vi "7HP_Process.vi"(0 "All samples in":sgl[][](array[numeric]), 1 "Serial number":u32, 2 "7HP Ch No":i16[](array[numeric]), 3 "Analysis info Index":i32[](array[numeric]), 4 "Probe Number":i32, 5 "Sampling Rate":dbl) -> ()   [LabVIEW 2021]
uses:
  <vilib>/Analysis/NI_AALBase.lvlib
  <vilib>/Analysis/baseanly.llb/Mean (DBL).vi
  Sub_vis/Upload Data.ctl
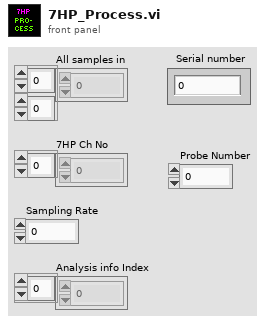
[diagram p1: front panel]
types:
  T1 = typedef "Upload Data.ctl" = enum16{"Voltage Array", "Time Trace Cluster"}
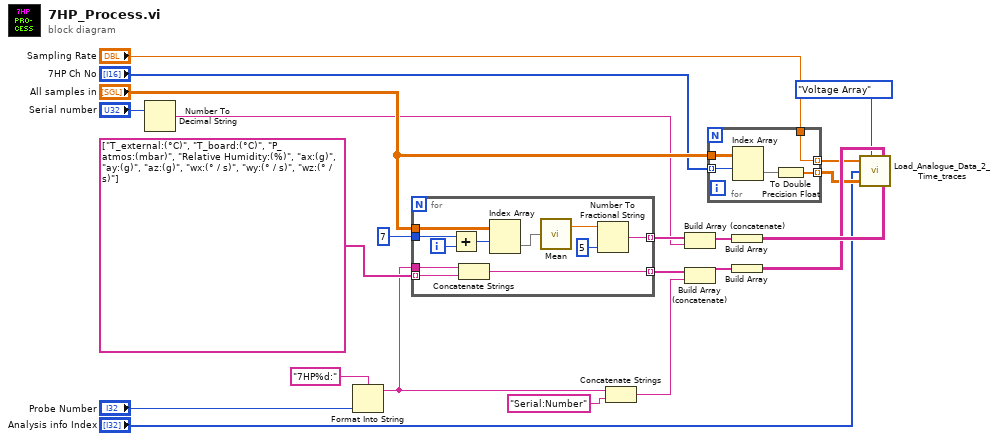
[diagram p0: block diagram]
diagram:
  n1 = Number To Decimal String(number="Serial number") -> (decimal integer string=w4:string)  [unwired: 1 in]
  n2 = Format Into String(format string="7HP%d:", "Probe Number") -> (resulting string=w9:string)  [unwired: 2 in, 1 out]
  n3 = for {
    tunnel: "All samples in" -> [w33]
    tunnel: 7 -> [w31]
    tunnel: w9 -> [w29]
    tunnel: string[] ["T_external:(°C)", "T_board:(°C)", "P_atmos:(mbar)", "Relative Humidity:(%)", "ax:(g)", "ay:(g)", "az:(g)", "wx:(° / s)", "wy:(° / s)", "wz:(° / s)"] -> [w28] mode=indexing
    tunnel: [w23] -> w10 mode=indexing
    tunnel: [w24] -> w7 mode=indexing
    i -> [w32]
    n4 = Add(x=w31, y=w32) -> (x+y=w30:i32)
    n5 = Concatenate Strings(w29, w28) -> (w24:string)
    n6 = Index Array(array=w33, index (row)=w30) -> (element=w27:sgl[])  [unwired: 1 in]
    n7 = call-poly <vilib>:"Mean.vi"("X"=w27) -> ("mean"=w26:dbl)  [unwired: 1 out]
    n8 = Number To Fractional String(number=w26, precision (6)=i16 5) -> (F-format string=w23:string)  [unwired: 2 in]
  }
  n9 = Concatenate Strings(w9, "Serial:Number") -> (w6:string)
  n10 = Build Array (concatenate)(w10, w4) -> (w3:string[])
  n11 = Build Array (concatenate)(w7, w6) -> (w5:string[])
  n12 = for {
    tunnel: "7HP Ch No" -> [w37] mode=indexing
    tunnel: "All samples in" -> [w38]
    tunnel: "Sampling Rate" -> [w34]
    tunnel: [w35] -> w15 mode=indexing
    tunnel: [w34] -> w16 mode=indexing
    n13 = Index Array(array=w38, index (row)=w37) -> (element=w36:sgl[])  [unwired: 1 in]
    n14 = To Double Precision Float(number=w36) -> (double precision float=w35:dbl[])
  }
  n15 = Build Array(w3) -> (w20:string[][])
  n16 = Build Array(w5) -> (w19:string[][])
  n17 = call "Load_Analogue_Data_2_Time_traces.vi"("Sampling Rate (Hz)"=w16, "Mode"=Upload_Data."Voltage Array", "Index"="Analysis info Index", "Voltage Array"=w15, "Metadata Names"=w19, "Metadata Values"=w20) -> ()  [unwired: 1 in]
